vi "post_run_times.vi"(8 "error in (no error)":errorcluster, 10 "Small?":bool, 11 "run_times":T1 caption="dcs_spot") -> (0 "error out":errorcluster)   [LabVIEW 2015]
doc: "Adds a new row to the dcs_spot table."
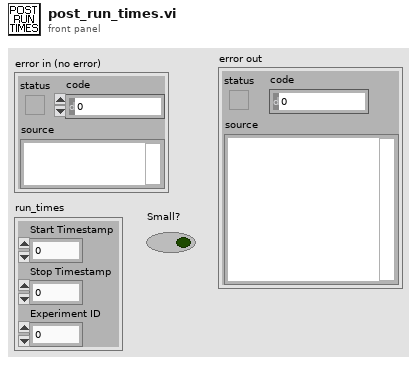
[diagram p1: front panel]
types:
  T1 = cluster{"Start Timestamp":i64, "Stop Timestamp":i64, "Experiment ID":i64}
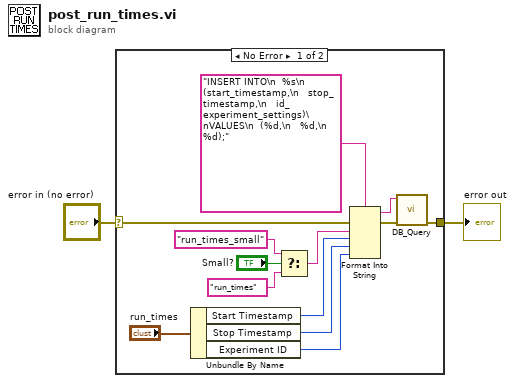
[diagram p0: block diagram]
diagram:
  n1 = case shown="No Error" "error in (no error)" {
    selector: "error in (no error)" -> [w14 w16]
    tunnel: [w7 w16] -> w1
    frame No Error {
      n2 = Unbundle By Name("run_times") -> ("Start Timestamp"=w11:i64, "Stop Timestamp"=w10:i64, "Experiment ID"=w9:i64)
      n3 = Select(t="run_times_small" ("Parameterized Query"), s="Small?", f="run_times" ("Parameterized Query")) -> (s? t:f=w3:string)
      n4 = Format Into String(format string="INSERT INTO\n  %s\n  (start_timestamp,\n   stop_timestamp,\n   id_experiment_settings)\nVALUES\n  (%d,\n   %d,\n   %d);" ("Parameterized Query"), error in=w14, w3, w11, w10, w9) -> (resulting string=w8:string, error out=w13:errorcluster)  [unwired: 1 in]
      n5 = call "DB_Query.vi"("error in (no error)"=w13, "Parameterized Query"=w8) -> ("error out"=w7:errorcluster)  [unwired: 7 in, 2 out]
    }
    frame Error {
    }
  }
  "error out" <- w1
